vi "genTask_fb_info_queue.vi"(8 "error in (no error)":errorcluster) -> (0 "error IO":errorcluster, 3 "pdbm_task_fb_info_queue":refnum<queue>)   [LabVIEW 2015, in "pdbm_task_route.lvlib"]
uses:
  pdbm_task_route.lvlib
  UsrDefine/TaskFeedbackCmd.ctl
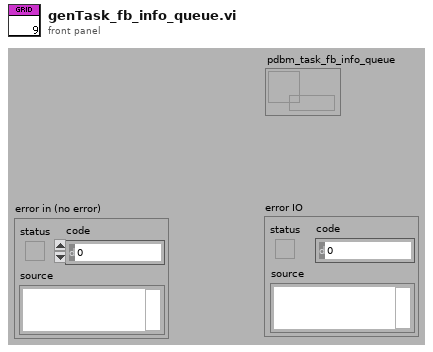
[diagram p1: front panel]
types:
  T1 = typedef "pdbm_task_route.lvlib/TaskFeedbackCmd.ctl" = cluster{"TaskRef":refnum<vi>, "Command":string, "Variant":variant}
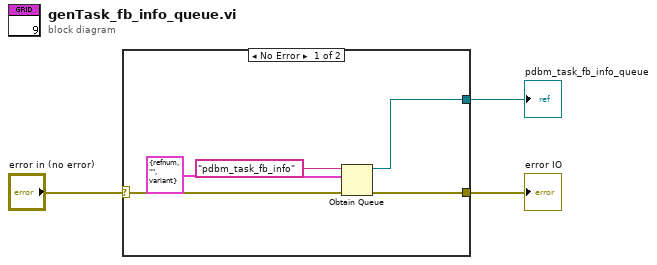
[diagram p0: block diagram]
diagram:
  n1 = case shown="No Error" "error in (no error)" {
    selector: "error in (no error)" -> [w8 w9]
    tunnel: [w5 _] -> w2
    tunnel: [w4 w9] -> w1
    frame No Error {
      n2 = Obtain Queue(name (unnamed)="pdbm_task_fb_info", element data type=T1 {"TaskRef"=refnum, "Command"="", "Variant"=variant} ("TaskFeedbackCmd"), error in (no error)=w8) -> (queue out=w5:refnum<queue>, error out=w4:errorcluster)  [unwired: 2 in, 1 out]
    }
    frame Error {
    }
  }
  "pdbm_task_fb_info_queue" <- w2
  "error IO" <- w1
